vi "Save File Sort Summary.vi"(8 "Error In":errorcluster, 10 "Summary Header":string[](array[string]), 11 "Input":string[][](array[string])) -> (0 "Error Out":errorcluster, 2 "Cycle Time Minutes":dbl, 3 "Output":string[][](array[string]))   [LabVIEW 2016]
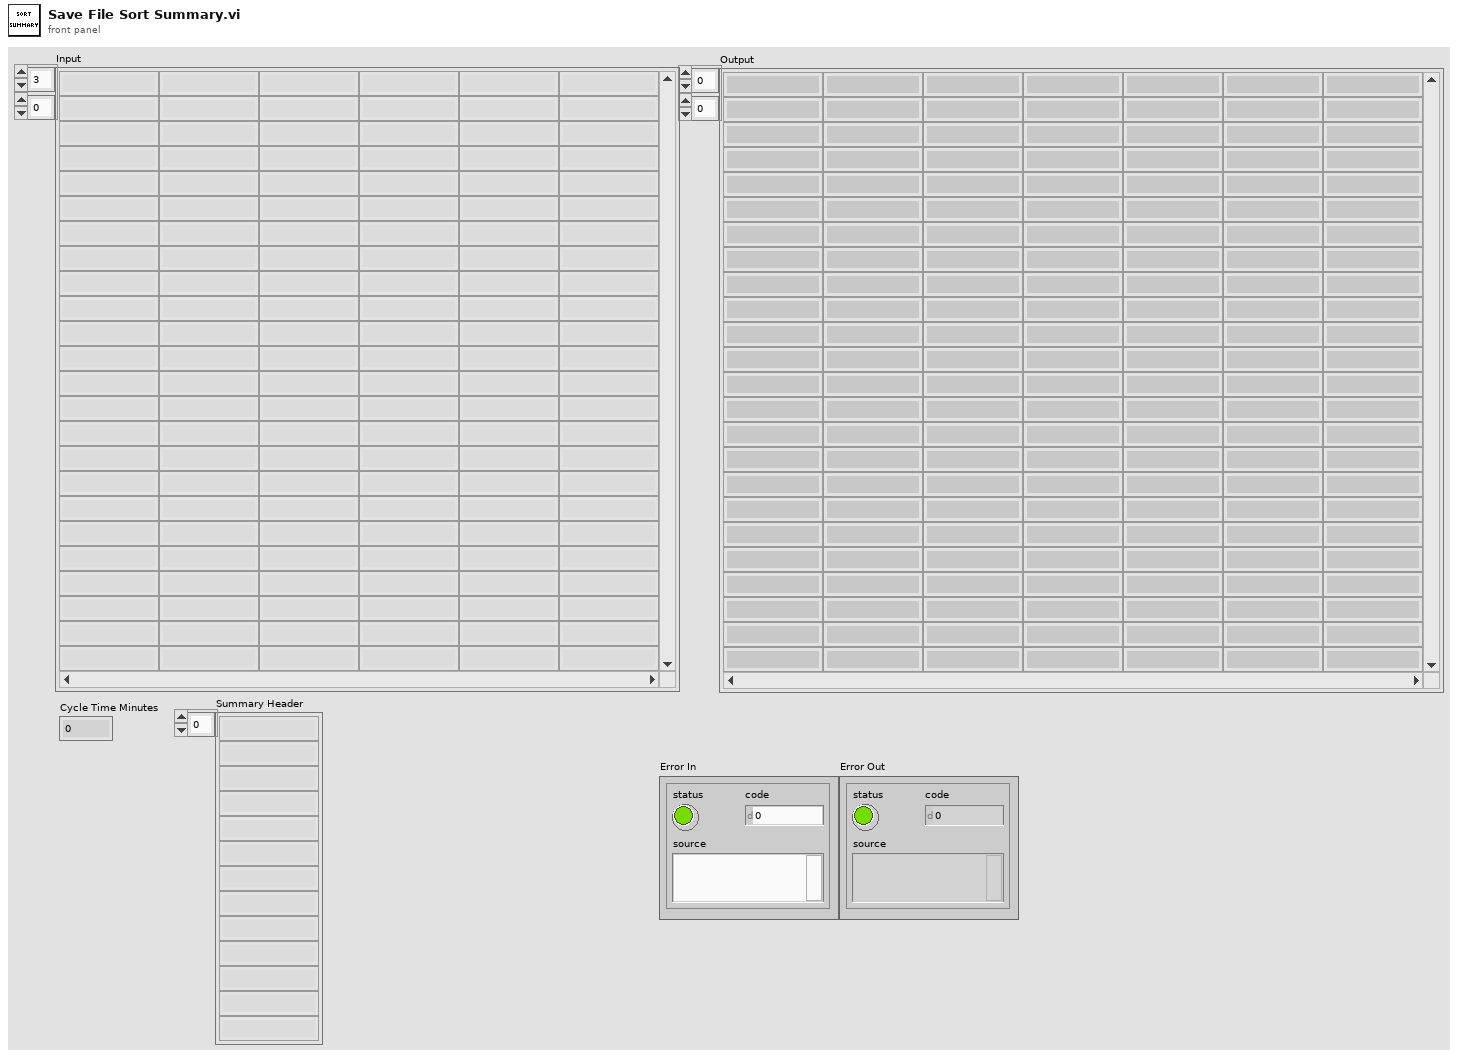
[diagram p1: front panel]
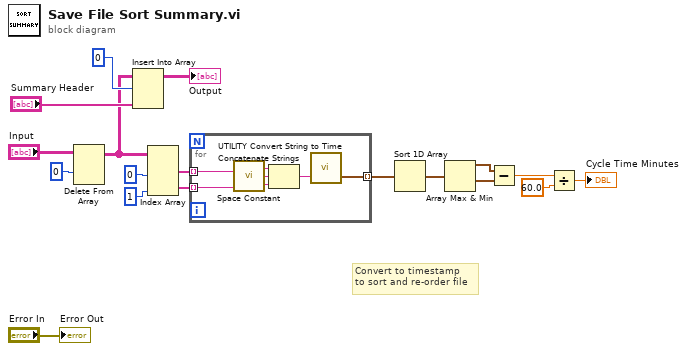
[diagram p0: block diagram]
diagram:
  # "Convert to timestamp\nto sort and re-order file"
  n1 = Delete From Array(array="Input", index (row)=0) -> (array with subset deleted=w2:string[][])  [unwired: 2 in, 1 out]
  n2 = Insert Into Array(array=w2, index (row)=0, new element="Summary Header") -> (→"Output":string[][])  [unwired: 1 in]
  n3 = Index Array(array=w2, index (col) #1=0 ("disabled index (col)"), index (col) #2=1 ("index (col)")) -> (element #1=w10:string[], element #2=w9:string[])  [unwired: 2 in]
  n4 = for {
    tunnel: w9 -> [w22] mode=indexing
    tunnel: w10 -> [w21] mode=indexing
    tunnel: [w19] -> w15 mode=indexing
    n5 = call <vilib>:"Space Constant.vi"() -> ("String"=w23:string)
    n6 = Concatenate Strings(w21, w23, w22) -> (w20:string)
    n7 = call "UTILITY Convert String to Time.vi"("date/time string"=w20) -> ("Resulting Time Stamp"=w19:timestamp)  [unwired: 8 in, 2 out]
  }
  n8 = Sort 1D Array(array=w15) -> (sorted array=w6:timestamp[])
  n9 = Array Max & Min(array=w6) -> (max value=w8:timestamp, min value=w7:timestamp)  [unwired: 2 out]
  n10 = Subtract(x=w8, y=w7) -> (x-y=w5:dbl)
  n11 = Divide(x=w5, y=60.0) -> (x/y=→"Cycle Time Minutes":dbl)
  "Error Out" <- "Error In"
